vi "Initialize_IconEditorSettings_Tree.vi"(8 "error in (no error)":errorcluster, 11 "Tree Refnum":refnum<vi>) -> (0 "error out":errorcluster)   [LabVIEW 2021, in "Settings.lvclass"]
uses:
  <resource>/plugins/NIIconEditor/Class/Settings/Settings.lvclass
panel:
  in  "Left Cell String 4":string="Text Tool"
  in  "Left Cell String 3":string="Layers"
  in  "Left Cell String 2":string="Templates"
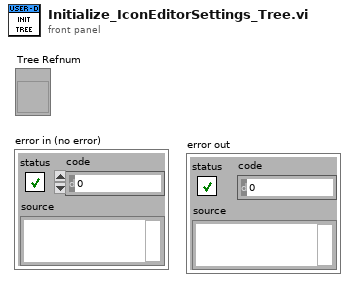
[diagram p1: front panel]
types:
  T1 = cluster{"Left Cell String":string, "Child Text":string[], "Child Tag":string, "Item Indent":i32, "Child Only?":bool, "Glyph Index":i32}[]
  T2 = cluster{"Left Cell String":string, "Child Text":string[], "Child Tag":string, "Item Indent":i32, "Child Only?":bool, "Glyph Index":i32}
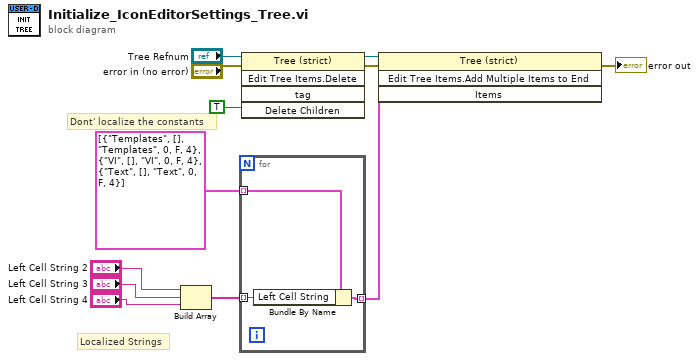
[diagram p0: block diagram]
diagram:
  # "Dont' localize the constants"
  # "Localized Strings"
  n1 = Build Array("Left Cell String 2", "Left Cell String 3", "Left Cell String 4") -> (w4:string[])
  n2 = for {
    tunnel: T1 [{"Left Cell String"="Templates", "Child Text"=[], "Child Tag"="Templates", "Item Indent"=0, "Child Only?"=FALSE, "Glyph Index"=4}, {"Left Cell String"="VI", "Child Text"=[], "Child Tag"="VI", "Item Indent"=0, "Child Only?"=FALSE, "Glyph Index"=4}, {"Left Cell String"="Text", "Child Text"=[], "Child Tag"="Text", "Item Indent"=0, "Child Only?"=FALSE, "Glyph Index"=4}] ("Items") -> [w15] mode=indexing
    tunnel: w4 -> [w14] mode=indexing
    tunnel: [w13] -> w3 mode=indexing
    n3 = Bundle By Name(cluster=w15, "Left Cell String"=w14) -> (w13:T2)
  }
  n4 = invoke on="Invoke Node" class="Tree (strict)" method="Edit Tree Items.Delete"(reference="Tree Refnum", error in="error in (no error)", "Delete Children"=TRUE ("Delete Children?")) -> (reference out=w9:refnum<vi>, error out=w11:errorcluster)  [unwired: 2 in, 3 out]
  n5 = invoke on="Invoke Node" class="Tree (strict)" method="Edit Tree Items.Add Multiple Items to End"(reference=w9, error in=w11, "Items"=w3) -> (error out=→"error out":errorcluster)  [unwired: 1 in, 3 out]
